vi "21-2.vi"() -> ()   [LabVIEW 2019, in "21.lvlib"]
uses:
  21.lvlib
panel:
  in  "Dice Positions":i32
  in  "Rolls Per Turn":i32
  out "Most Wins":u64
  in  "Score To Win":i32=21
  in  "Number of Positions":i32=10
  out "P2 Wins":u64
  out "P1 Wins":u64
  in  "Sample?":bool
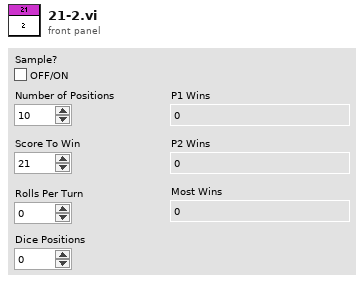
[diagram p1: front panel]
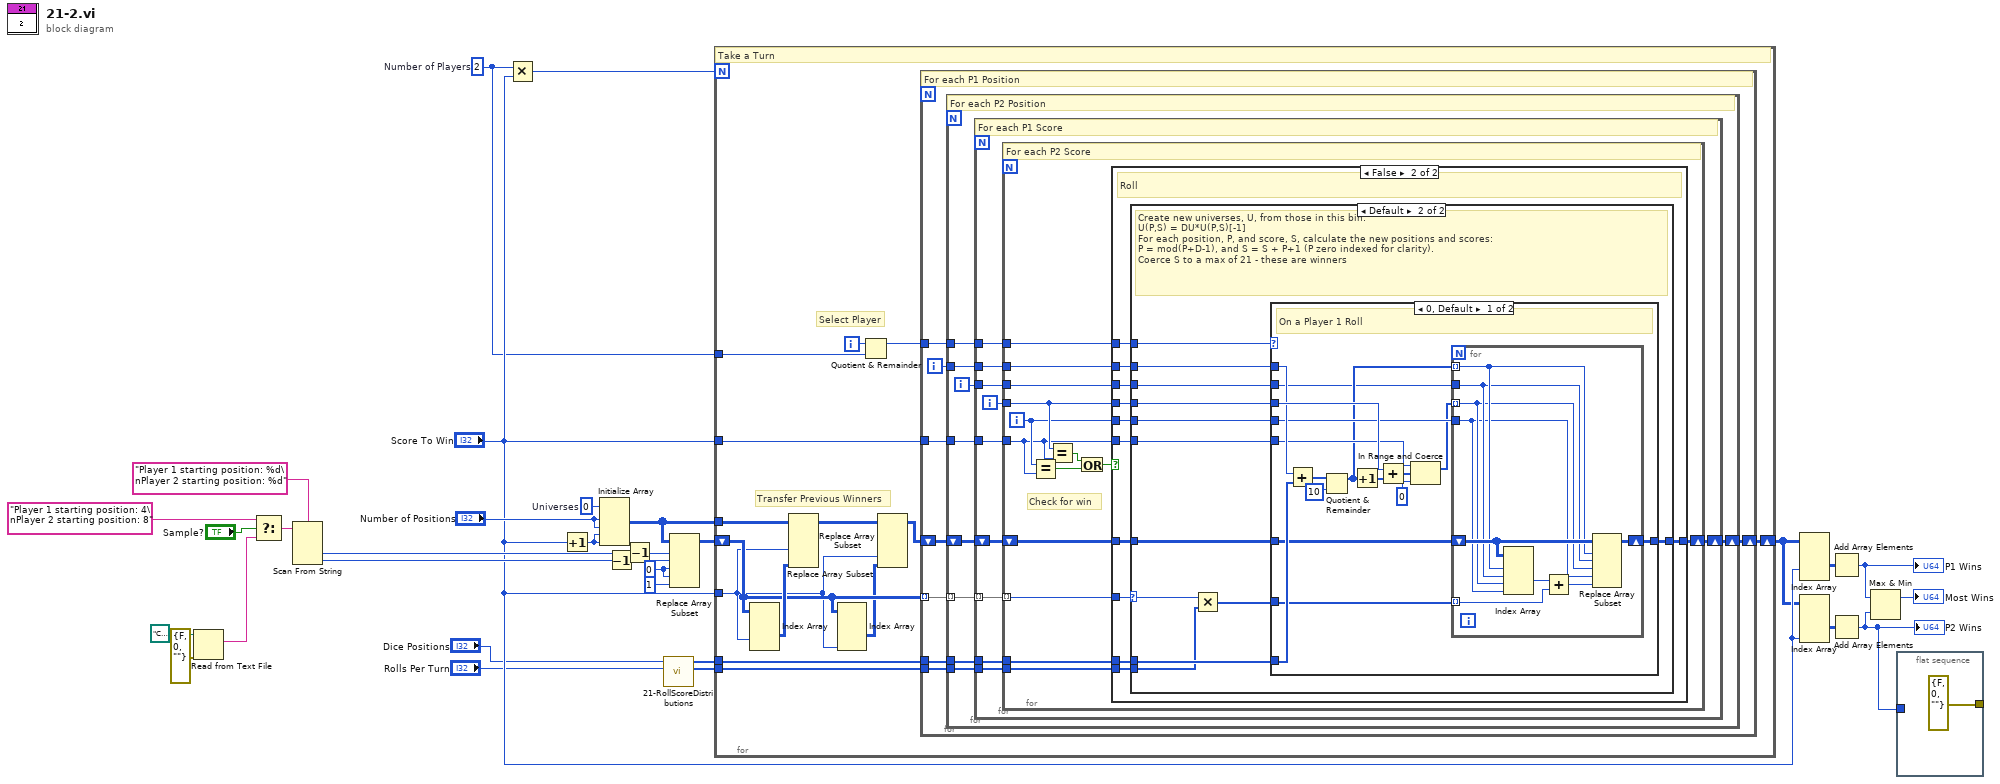
[diagram p0: block diagram]
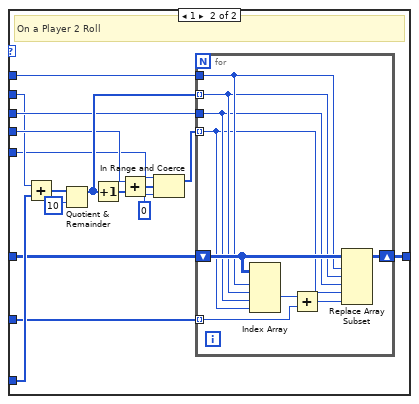
[diagram p4: hidden frame]
diagram:
  w7 = 2  # Number of Players
  w21 = u64 0  # Universes
  w17 = 0 ("index (row)")
  n1 = Read from Text File(file (use dialog)=path "C:/Users/craig.walker/Documents/GitHub/lv2019-Advent-of-Code-2021/21/input.txt", error in=errorcluster {"status"=FALSE, "code"=0, "source"=""}) -> (text=w28:string)  [unwired: 2 in, 3 out]
  n2 = Select(t="Player 1 starting position: 4\nPlayer 2 starting position: 8", s="Sample?", f=w28) -> (s? t:f=w30:string)
  n3 = Scan From String(format string="Player 1 starting position: %d\nPlayer 2 starting position: %d", input string=w30) -> (output 1=w18:i32, output 2=w24:i32)  [unwired: 4 in, 3 out]
  n4 = Multiply(x=w7, y="Score To Win") -> (x*y=w14:i32)
  n5 = Increment(x="Score To Win") -> (x+1=w22:i32)
  n6 = Initialize Array(w21, "Number of Positions", "Number of Positions", w22, w22) -> (w23:u64[][][][])
  n7 = Decrement(x=w24) -> (x-1=w15:i32)
  n8 = Decrement(x=w18) -> (x-1=w16:i32)
  n9 = call "21-RollScoreDistributions.vi"("Rolls Per Turn"="Rolls Per Turn", "Dice Positions"="Dice Positions") -> ("DU"=w3:u64[], "D"=w4:u64[])  [unwired: 8 in]
  n10 = Replace Array Subset(array=w23, new element=u64 1 ("index (row)"), index (dim 0)=w16, index (dim 1)=w15, index (dim 2)=w17, index (dim 3)=w17) -> (w25:u64[][][][])
  n11 = for {
    N: w14 -> [_]
    tunnel: w4 -> [w45]
    tunnel: w3 -> [w43]
    tunnel: w23 -> [w41]
    shift-right: [w34] -> w8
    shift-left: w25 -> [w37]
    tunnel: "Score To Win" -> [w42]
    tunnel: "Score To Win" -> [w35]
    tunnel: w7 -> [w33]
    i -> [w44]
    # "Select Player"
    # "Transfer Previous Winners"
    # "Take a Turn"
    n12 = Index Array(array=w37, index (dim 2)=w35) -> (element=w40:u64[][][])  [unwired: 3 in]
    n13 = Replace Array Subset(array=w41, new element=w40, index (dim 2)=w35) -> (w39:u64[][][][])  [unwired: 3 in]
    n14 = Index Array(array=w37, index (dim 3)=w35) -> (element=w36:u64[][][])  [unwired: 3 in]
    n15 = Quotient & Remainder(x=w44, y=w33) -> (x-y*floor(x/y)=w32:i32)  [unwired: 1 out]
    n16 = Replace Array Subset(array=w39, new element=w36, index (dim 3)=w35) -> (w38:u64[][][][])  [unwired: 3 in]
    n17 = for {
      tunnel: w37 -> [w53] mode=indexing
      tunnel: w45 -> [w52]
      tunnel: w32 -> [w51]
      tunnel: w43 -> [w50]
      shift-right: [w48] -> w34
      shift-left: w38 -> [w49]
      tunnel: w42 -> [w46]
      i -> [w47]
      # "For each P1 Position"
      n18 = for {
        tunnel: w53 -> [w57] mode=indexing
        tunnel: w52 -> [w62]
        tunnel: w51 -> [w56]
        tunnel: w50 -> [w60]
        shift-right: [w58] -> w48
        shift-left: w49 -> [w59]
        tunnel: w47 -> [w55]
        tunnel: w46 -> [w54]
        i -> [w61]
        # "For each P2 Position"
        n19 = for {
          tunnel: w57 -> [w67] mode=indexing
          tunnel: w62 -> [w72]
          tunnel: w56 -> [w66]
          tunnel: w61 -> [w71]
          tunnel: w60 -> [w64]
          shift-right: [w68] -> w58
          shift-left: w59 -> [w69]
          tunnel: w55 -> [w65]
          tunnel: w54 -> [w63]
          i -> [w70]
          # "For each P1 Score"
          n20 = for {
            tunnel: w72 -> [w86]
            tunnel: w71 -> [w85]
            tunnel: w70 -> [w78]
            tunnel: w67 -> [w82] mode=indexing
            tunnel: w66 -> [w81]
            shift-right: [w83] -> w68
            shift-left: w69 -> [w84]
            tunnel: w65 -> [w80]
            tunnel: w64 -> [w79]
            tunnel: w63 -> [w73]
            i -> [w77]
            # "Check for win"
            # "For each P2 Score"
            n21 = Equal?(x=w77, y=w73) -> (x = y?=w76:bool)
            n22 = Equal?(x=w78, y=w73) -> (x = y?=w75:bool)
            n23 = Or(x=w75, y=w76) -> (x .or. y?=w74:bool)
            n24 = case shown="False" w74 {
              tunnel: w86 -> [_ w98]
              tunnel: w85 -> [_ w97]
              tunnel: w78 -> [_ w96]
              tunnel: w84 -> [w87 w95]
              tunnel: [w87 w94] -> w83
              tunnel: w82 -> [_ w93]
              tunnel: w81 -> [_ w92]
              tunnel: w80 -> [_ w91]
              tunnel: w79 -> [_ w89]
              tunnel: w73 -> [_ w88]
              tunnel: w77 -> [_ w90]
              frame True {
                # "This bin is already a winner, winners transferred at start U(P,SWin) = U(P,SWin)[-1]"
              }
              frame False {
                # "Roll"
                n25 = case shown="Default" w93 {
                  selector: w93 -> [_ w101]
                  tunnel: w98 -> [_ w111]
                  tunnel: w97 -> [_ w104]
                  tunnel: w96 -> [_ w107]
                  tunnel: w95 -> [w99 w109]
                  tunnel: [w99 w110] -> w94
                  tunnel: w92 -> [_ w105]
                  tunnel: w91 -> [_ w106]
                  tunnel: w90 -> [_ w108]
                  tunnel: w89 -> [_ w103]
                  tunnel: w88 -> [_ w100]
                  frame 0 {
                    # "no universes, U=0"
                  }
                  frame Default {
                    # "Create new universes, U, from those in this bin:\nU(P,S) = DU*U(P,S)[-1]\nFor each position, P, and score, S, calculate the new positions and scores:\nP = mod(P+D-1), and S = S + P+1 (P zero indexed for clarity).\nCoerce S to a max of 21 - these are winners"
                    n26 = Multiply(x=w101, y=w103) -> (x*y=w102:u64[])
                    n27 = case shown="0, Default" w105 {
                      tunnel: w111 -> [w127 w152]
                      tunnel: [w124 w148] -> w110
                      tunnel: w109 -> [w123 w147]
                      tunnel: w108 -> [w120 w143]
                      tunnel: w107 -> [w122 w144]
                      tunnel: w106 -> [w121 w141]
                      tunnel: w104 -> [w112 w142]
                      tunnel: w102 -> [w119 w145]
                      tunnel: w100 -> [w115 w137]
                      frame 0, Default {
                        # "On a Player 1 Roll"
                        n28 = Add(x=w121, y=w127) -> (x+y=w126:u64[])
                        n29 = Quotient & Remainder(x=w126, y=10) -> (x-y*floor(x/y)=w114:u64[])  [unwired: 1 out]
                        n30 = Increment(x=w114) -> (x+1=w113:u64[])
                        n31 = Add(x=w122, y=w113) -> (x+y=w117:u64[])
                        n32 = In Range and Coerce(upper limit=w115, x=w117, lower limit=0) -> (coerced(x)=w116:u64[])  [unwired: 1 out]
                        n33 = for {
                          shift-right: [w136] -> w124
                          shift-left: w123 -> [w135]
                          tunnel: w116 -> [w131] mode=indexing
                          tunnel: w114 -> [w133] mode=indexing
                          tunnel: w120 -> [w130]
                          tunnel: w112 -> [w132]
                          tunnel: w119 -> [w128] mode=indexing
                          n34 = Index Array(array=w135, index (dim 0)=w133, index (dim 1)=w132, index (dim 2)=w131, index (dim 3)=w130) -> (element=w134:u64)
                          n35 = Add(x=w134, y=w128) -> (x+y=w129:u64)
                          n36 = Replace Array Subset(array=w135, new element=w129, index (dim 0)=w133, index (dim 1)=w132, index (dim 2)=w131, index (dim 3)=w130) -> (w136:u64[][][][])
                        }
                      }
                      frame 1 {
                        # "On a Player 2 Roll"
                        n37 = Add(x=w142, y=w152) -> (x+y=w151:u64[])
                        n38 = Quotient & Remainder(x=w151, y=10) -> (x-y*floor(x/y)=w146:u64[])  [unwired: 1 out]
                        n39 = Increment(x=w146) -> (x+1=w149:u64[])
                        n40 = Add(x=w143, y=w149) -> (x+y=w139:u64[])
                        n41 = In Range and Coerce(upper limit=w137, x=w139, lower limit=0) -> (coerced(x)=w138:u64[])  [unwired: 1 out]
                        n42 = for {
                          shift-right: [w161] -> w148
                          shift-left: w147 -> [w160]
                          tunnel: w138 -> [w155] mode=indexing
                          tunnel: w146 -> [w157] mode=indexing
                          tunnel: w144 -> [w156]
                          tunnel: w141 -> [w158]
                          tunnel: w145 -> [w153] mode=indexing
                          n43 = Index Array(array=w160, index (dim 0)=w158, index (dim 1)=w157, index (dim 2)=w156, index (dim 3)=w155) -> (element=w159:u64)
                          n44 = Add(x=w159, y=w153) -> (x+y=w154:u64)
                          n45 = Replace Array Subset(array=w160, new element=w154, index (dim 0)=w158, index (dim 1)=w157, index (dim 2)=w156, index (dim 3)=w155) -> (w161:u64[][][][])
                        }
                      }
                    }
                  }
                }
              }
            }
          }
        }
      }
    }
  }
  n46 = Index Array(array=w8, index (dim 2)="Score To Win") -> (element=w11:u64[][][])  [unwired: 3 in]
  n47 = Index Array(array=w8, index (dim 3)="Score To Win") -> (element=w10:u64[][][])  [unwired: 3 in]
  n48 = Add Array Elements(numeric array=w11) -> (sum=w9:u64)
  "P1 Wins" <- w9
  n49 = Add Array Elements(numeric array=w10) -> (sum=w1:u64)
  "P2 Wins" <- w1
  n50 = Max & Min(x=w9, y=w1) -> (max(x,y)=→"Most Wins":u64)  [unwired: 1 out]
  n51 = flat-sequence {
    tunnel: w1 -> [_]
    tunnel: [errorcluster {"status"=FALSE, "code"=0, "source"=""} ("error constant")] -> _
    frame #0 {
    }
  }
